vi "fgv_Functional Param.vi"() -> ()   [LabVIEW 2020]
uses:
  Typedefs/Controls/Functional Parameters.ctl
panel:
  in  "Functional_Enum":enum16{"Initialize", "write", "read"}(ring)
  in  "Functional Settings":T1={"AOL Mode"=enum."", "FrameSize"=0.0, "GridXY"=1.0, "GridZ"=1.0, "DAQ Length (sec)"=0.2, "No of Trials"=0.0, "TrigDelay\n(Sec)"=1.0, "AOD fill"=0.0, "Cycles"=0.0}
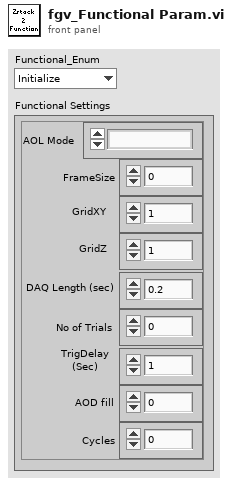
[diagram p1: front panel]
types:
  T1 = typedef "Functional Parameters.ctl" = cluster{"AOL Mode":enum16{""}, "FrameSize":dbl, "GridXY":dbl, "GridZ":dbl, "DAQ Length (sec)":sgl, "No of Trials":dbl, "TrigDelay\n(Sec)":dbl, "AOD fill":dbl, "Cycles":dbl}
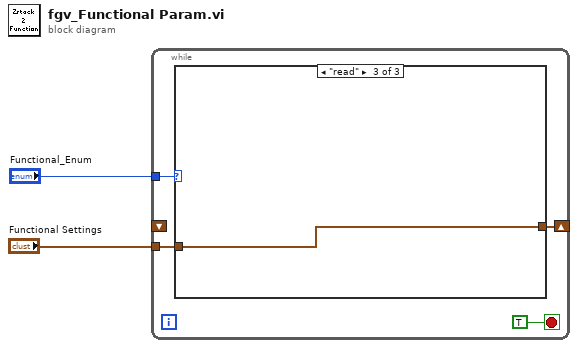
[diagram p0: block diagram]
diagram:
  n1 = while {
    tunnel: "Functional Settings" -> [w4]
    shift-right: [w5] -> _
    shift-left: _ -> [_]
    tunnel: "Functional_Enum" -> [w3]
    stop <- TRUE stop-if-true
    n2 = case shown="\"read\"" w3 {
      tunnel: [w7 w8 w9] -> w5
      tunnel: w4 -> [w7 w8 w9]
      frame "Initialize", Default {
      }
      frame "write" {
      }
      frame "read" {
      }
    }
  }
